vi "readTemperature__.vi"(8 "error in (no error)":errorcluster, 11 "OvenController in":refnum<class "OvenController.lvclass">) -> (0 "error out":errorcluster, 2 "temperature[°C]":i32, 3 "OvenController out":refnum<class "OvenController.lvclass">)   [LabVIEW 2023, in "AbstractFactory.lvlib" / "OvenController.lvclass"]
uses:
  OvenController.lvclass
  OvenController.lvclass/OvenController.ctl
  IResponseParser/IResponseParser.lvclass
  IConnection/IConnection.lvclass
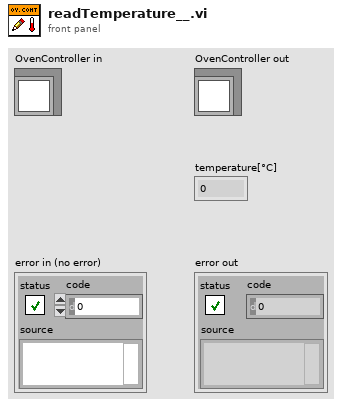
[diagram p1: front panel]
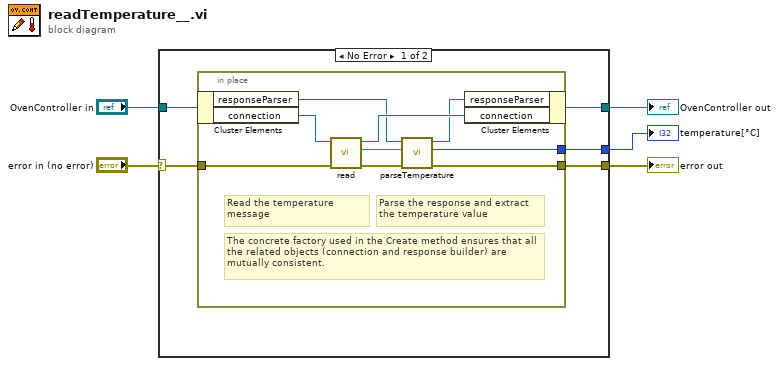
[diagram p0: block diagram]
diagram:
  n1 = case shown="No Error" "error in (no error)" {
    selector: "error in (no error)" -> [w8 w21]
    tunnel: [w7 w21] -> w4
    tunnel: [w10 w20] -> w2
    tunnel: "OvenController in" -> [w9 w20]
    tunnel: [w6 _] -> w1
    frame No Error {
      n2 = in-place {
        in-place-border: w8 -> [w17]
        in-place-border: [w11] -> w7
        in-place-border: [w16] -> w6
        # "The concrete factory used in the Create method ensures that all the related objects (connection and response builder) are mutually consistent."
        # "Parse the response and extract the temperature value"
        # "Read the temperature message"
        n3 = in-place-cluster #1(w9) -> ("responseParser"=w13:refnum<class "IResponseParser.lvclass">, "connection"=w19:refnum<class "IConnection.lvclass">)
        n4 = call-dynamic "read.vi"("error in (no error)"=w17, "IConnection in"=w19) -> ("error out"=w15:errorcluster, "message"=w14:string, "IConnection out"=w18:refnum<class "IConnection.lvclass">)  [unwired: 7 in]
        n5 = call-dynamic "parseTemperature.vi"("error in (no error)"=w15, "response"=w14, "IResponseParser in"=w13) -> ("error out"=w11:errorcluster, "temperature"=w16:i32, "IResponseParser out"=w12:refnum<class "IResponseParser.lvclass">)  [unwired: 6 in]
        n6 = in-place-cluster #1("responseParser"=w12, "connection"=w18) -> (w10:refnum<class "OvenController.lvclass">)
      }
    }
    frame Error {
    }
  }
  "error out" <- w4
  "OvenController out" <- w2
  "temperature[°C]" <- w1
